vi "Read Person.vi"(8 "error in (no error)":errorcluster, 11 "Person Test in":refnum<class "Person Test.lvclass">) -> (0 "error out":errorcluster, 2 "Person.lvclass":refnum<class "Person.lvclass">, 3 "Person Test out":refnum<class "Person Test.lvclass">)   [LabVIEW 2020, in "Person Test.lvclass"]
uses:
  Person Test.lvclass
  Person Test.lvclass/Person Test.ctl
  Processes/People/Person/Person.lvclass
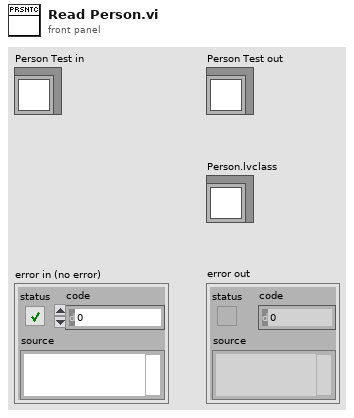
[diagram p1: front panel]
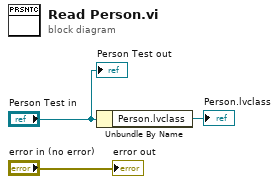
[diagram p0: block diagram]
diagram:
  n1 = Unbundle By Name("Person Test in") -> ("Person.lvclass"=→"Person.lvclass":refnum<class "Person.lvclass">)
  "Person Test out" <- "Person Test in"
  "error out" <- "error in (no error)"
